vi "CalculateMcsaLowRateFeatures.vi"(5 "Motor Info":T4, 7 "Channel Phasors":T5[](array[typedef]), 8 "error in (no error)":errorcluster, 9 "data flow map in":T10, 10 "waveforms":waveform(sgl)[](array[waveform]), 11 "Channels":T6[](array[typedef])) -> (0 "error out":errorcluster, 2 "Calculation Cache":T1, 3 "Channels":T6[](array[typedef]))   [LabVIEW 2017, in "McsaAnalysisFunctions.lvlib"]
uses:
  <vilib>/addons/InsightCM/Utilities/Analysis/MCSA/McsaAnalysisFunctions.lvlib
  <vilib>/addons/PointValueMap/controls/PointMap.ctl
  <vilib>/addons/InsightCM/Utilities/Analysis/MCSA/controls/McsaChannel.ctl
  <vilib>/addons/InsightCM/Utilities/Analysis/Shared/controls/Feature.ctl
  <vilib>/addons/InsightCM/Utilities/Analysis/Shared/controls/AmplitudeScale.ctl
  <vilib>/addons/InsightCM/MessageBus/Base/controls/KeyValuePair.ctl
  <vilib>/addons/InsightCM/Utilities/Analysis/MCSA/controls/McsaChannelPhasor.ctl
  <vilib>/addons/InsightCM/Utilities/Analysis/MCSA/controls/McsaMotor.ctl
  <vilib>/addons/InsightCM/Utilities/Analysis/MCSA/controls/MotorCalculationCache.ctl
  <vilib>/addons/Electrical Power/Basic/Measurement/subVIs/basic_Power Value.ctl
  <vilib>/addons/InsightCM/Utilities/Analysis/MCSA/controls/TorqueLoadEfficiency.ctl
  <vilib>/addons/InsightCM/Utilities/Analysis/MCSA/controls/PowerSpectrumCalculationCache.ctl
  <vilib>/addons/_NISVFA/_Shared subVIs/Controls/svc_Spectrum Info.ctl
  <vilib>/addons/_NISVFA/_Shared subVIs/Controls/svc_X-Axis Units.ctl
  <vilib>/addons/_NISVFA/_Shared subVIs/Controls/svc_Spectrum Type.ctl
  <vilib>/addons/_NISVFA/_Shared subVIs/Controls/svc_Engineering Units Text Ring.ctl
  <vilib>/addons/_NISVFA/_Shared subVIs/Controls/svc_Weighting Filter Text Ring.ctl
  <vilib>/addons/_NISVFA/_Shared subVIs/Controls/svc_Complimentary Spectrum Units.ctl
  <vilib>/addons/Electrical Power/Basic/NI_EP_Basic.lvlib
  <vilib>/addons/PointValueMap/PointValueMap.lvlib
  <vilib>/addons/InsightCM/Utilities/MCSA/McsaUtilities.lvlib
  <vilib>/addons/InsightCM/Utilities/Analysis/Shared/AnalysisHelper.lvlib
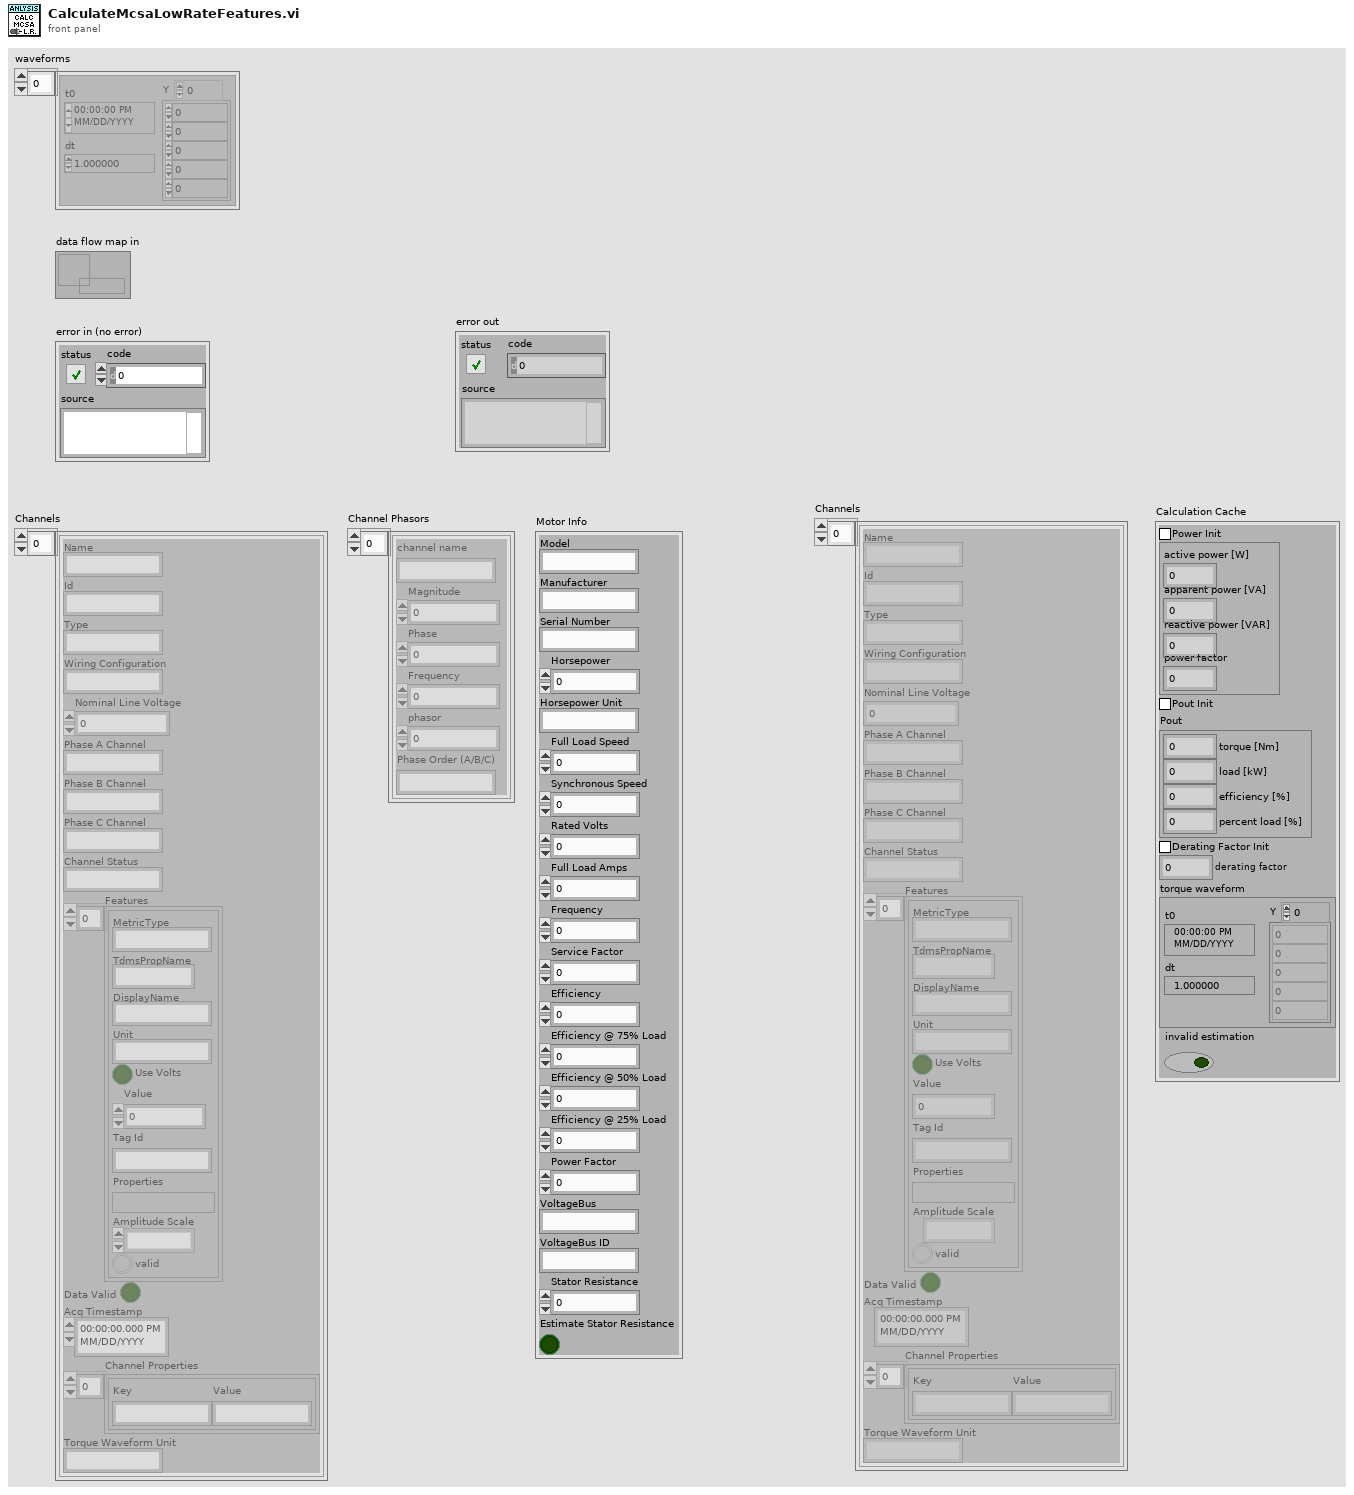
[diagram p1: front panel]
types:
  T1 = typedef "McsaAnalysisFunctions.lvlib/MotorCalculationCache.ctl" = cluster{"Power Init":bool, "power value":T2, "Pout Init":bool, "Pout":T3, "Derating Factor Init":bool, "derating factor":sgl, "torque waveform":waveform(dbl), "invalid estimation":bool}
  T2 = typedef "NI_EP_Basic.lvlib/basic_Power Value.ctl" = cluster{"active power [W]":dbl, "apparent power [VA]":dbl, "reactive power [VAR]":dbl, "power factor":dbl}
  T3 = typedef "McsaAnalysisFunctions.lvlib/TorqueLoadEfficiency.ctl" = cluster{"torque [Nm]":dbl, "load [kW]":dbl, "efficiency [%]":dbl, "percent load [%]":dbl}
  T4 = typedef "McsaAnalysisFunctions.lvlib/McsaMotor.ctl" = cluster{"Model":string, "Manufacturer":string, "Serial Number":string, "Horsepower":dbl, "Horsepower Unit":string, "Full Load Speed":dbl, "Synchronous Speed":dbl, "Rated Volts":dbl, "Full Load Amps":dbl, "Frequency":dbl, "Service Factor":dbl, "Efficiency":dbl, "Efficiency @ 75% Load":dbl, "Efficiency @ 50% Load":dbl, "Efficiency @ 25% Load":dbl, "Power Factor":dbl, "VoltageBus":string, "VoltageBus ID":string, "Stator Resistance":dbl, "Estimate Stator Resistance":bool}
  T5 = typedef "McsaAnalysisFunctions.lvlib/McsaChannelPhasor.ctl" = cluster{"channel name":string, "Magnitude":dbl, "Phase":dbl, "Frequency":dbl, "phasor":cdb, "Phase Order (A/B/C)":string}
  T6 = typedef "McsaAnalysisFunctions.lvlib/McsaChannel.ctl" = cluster{"Name":string, "Id":string, "Type":string, "Wiring Configuration":string, "Nominal Line Voltage":dbl, "Phase A Channel":string, "Phase B Channel":string, "Phase C Channel":string, "Channel Status":string, "Features":T7[], "Data Valid":bool, "Acq Timestamp":timestamp, "Channel Properties":T9[], "Torque Waveform Unit":string}
  T7 = typedef "AnalysisHelper.lvlib/Feature.ctl" = cluster{"MetricType":string, "TdmsPropName":string, "DisplayName":string, "Unit":string, "Use Volts":bool, "Value":dbl, "Tag Id":string, "Properties":variant, "Amplitude Scale":T8, "valid":bool}
  T8 = typedef "AnalysisHelper.lvlib/AmplitudeScale.ctl" = enum16{"rms", "peak", "pk-pk"}
  T9 = typedef "KeyValuePair.ctl" = cluster{"Key":string, "Value":string}
  T10 = typedef "PointValueMap.lvlib/PointMap.ctl" = refnum<data-value>
  T11 = typedef "McsaAnalysisFunctions.lvlib/PowerSpectrumCalculationCache.ctl" = cluster{"Spectrum Init":bool, "Power Spectrum":cluster{"f0":dbl, "df":dbl, "magnitude":dbl[]}, "spectrum info":T12}
  T12 = typedef "svc_Spectrum Info.ctl" = cluster{"channel name":string, "description":string, "x-axis units":T13, "spectral info":cluster{"spectrum type":T14, "linear/dB":enum16{"linear", "dB"}, "window":u16, "window size":i32, "FFT size":i32}, "engineering units":T15, "custom label":string, "dB reference [EU]":dbl, "peak units":enum16{"rms", "peak", "peak-peak"}, "weighting filter":T16, "spectral density?":bool, "unit label":string, "spectrum skewed?":bool, "complimentary spectrum units":T17}
  T13 = typedef "svc_X-Axis Units.ctl" = u16
  T14 = typedef "svc_Spectrum Type.ctl" = enum16{"FFT Spectrum [complex]", "Amplitude [Magnitude]", "Power [Magnitude^2]", "Cross Spectrum [complex]", "Frequency Response [Complex]"}
  T15 = typedef "svc_Engineering Units Text Ring.ctl" = u16
  T16 = typedef "svc_Weighting Filter Text Ring.ctl" = u16
  T17 = typedef "svc_Complimentary Spectrum Units.ctl" = enum16{"none", "radians", "degrees", "cycles", "imaginary"}
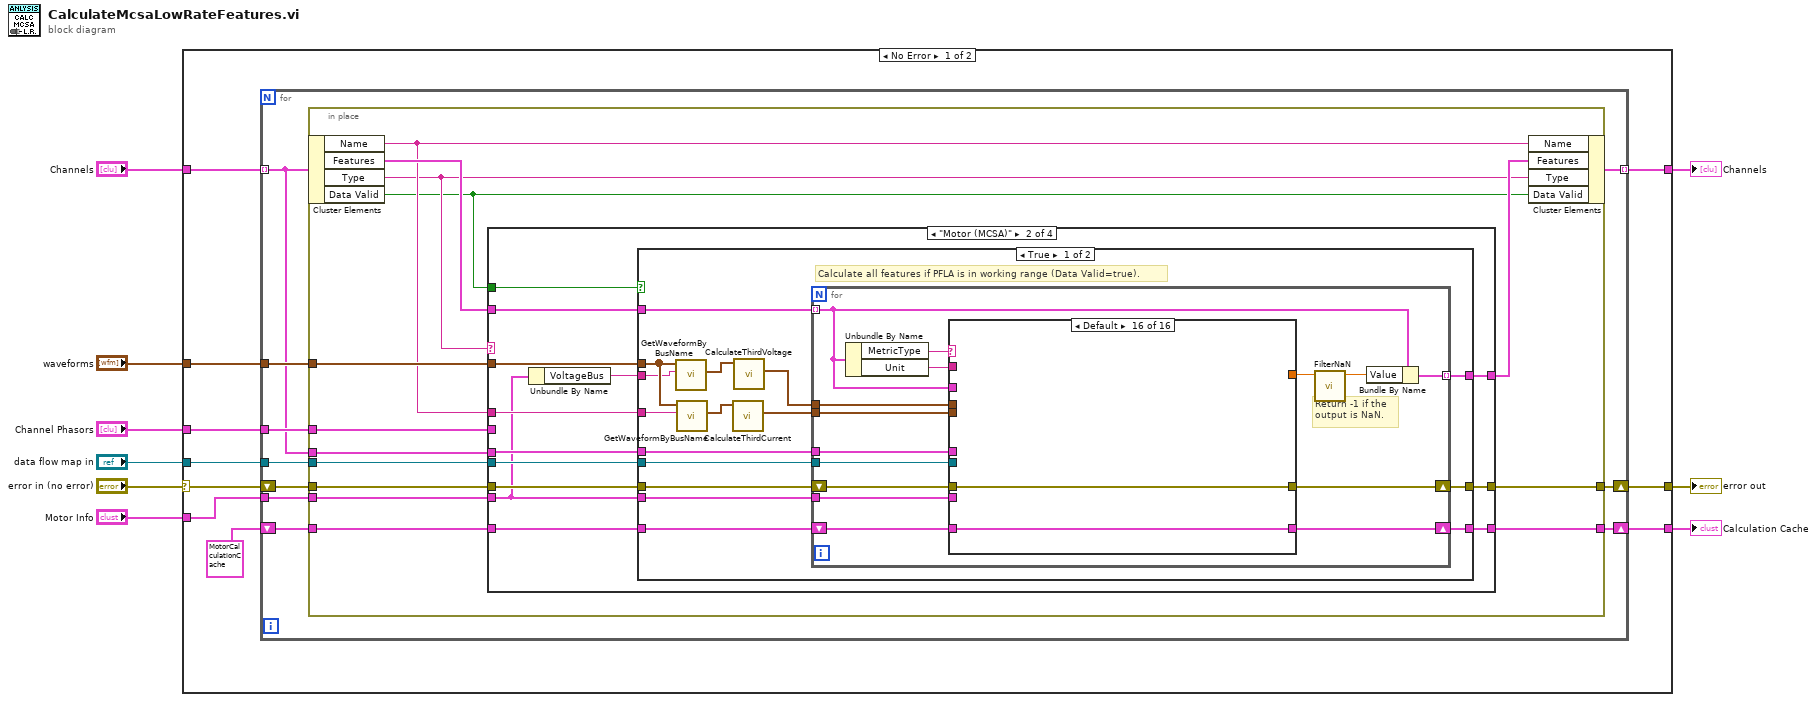
[diagram p0: block diagram]
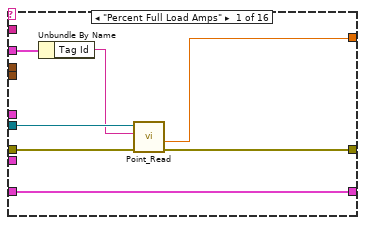
[diagram p3: hidden frame]
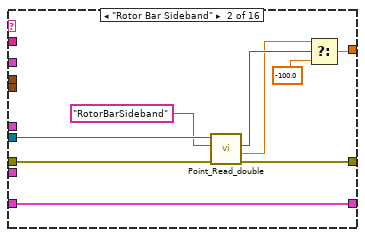
[diagram p4: hidden frame]
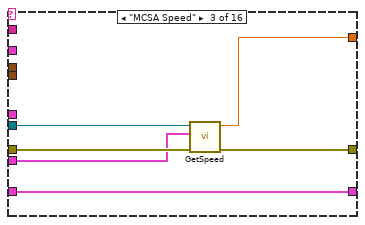
[diagram p5: hidden frame]
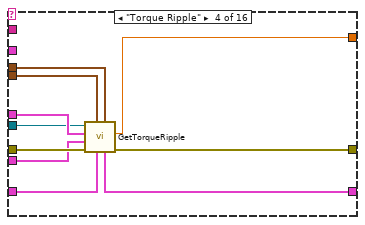
[diagram p6: hidden frame]
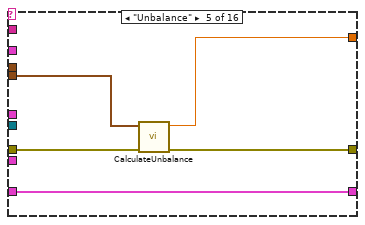
[diagram p7: hidden frame]
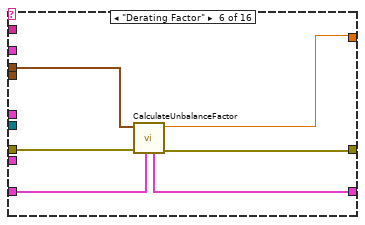
[diagram p8: hidden frame]
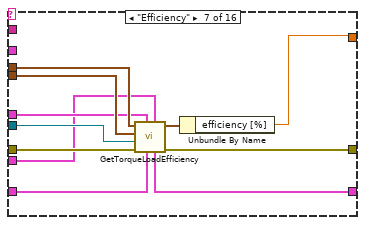
[diagram p9: hidden frame]
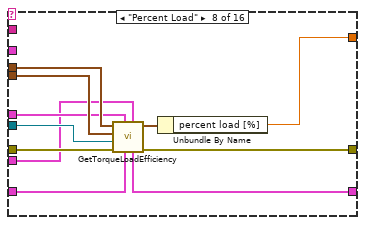
[diagram p10: hidden frame]
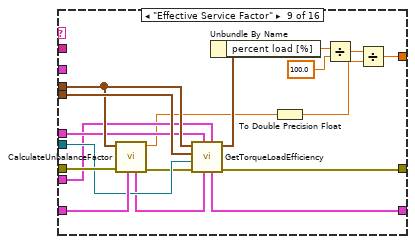
[diagram p11: hidden frame]
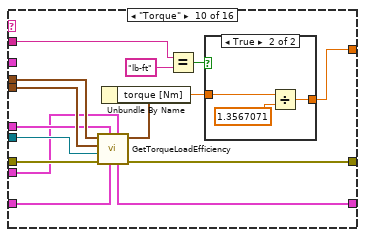
[diagram p12: hidden frame]
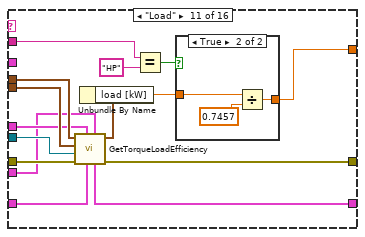
[diagram p14: hidden frame]
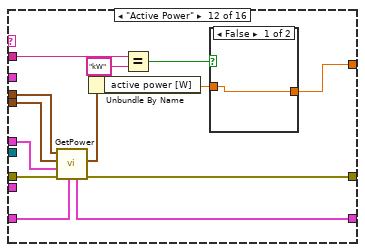
[diagram p16: hidden frame]
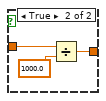
[diagram p17: hidden frame]
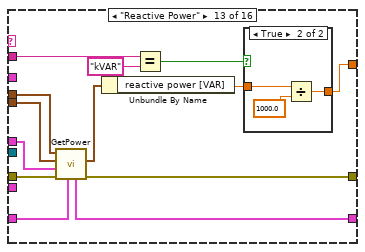
[diagram p18: hidden frame]
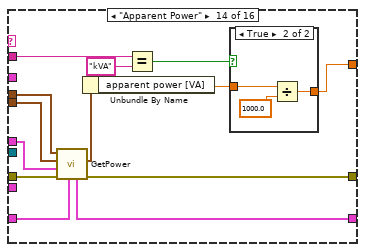
[diagram p20: hidden frame]
diagram:
  n1 = case shown="No Error" "error in (no error)" {
    selector: "error in (no error)" -> [w19 w402]
    tunnel: [w17 w402] -> w9
    tunnel: "waveforms" -> [w18 _]
    tunnel: "data flow map in" -> [w16 _]
    tunnel: "Channels" -> [w15 w401]
    tunnel: [w14 w401] -> w4
    tunnel: "Channel Phasors" -> [w13 _]
    tunnel: "Motor Info" -> [w12 _]
    tunnel: [w11 _] -> w1
    frame No Error {
      n2 = for {
        tunnel: w15 -> [w22] mode=indexing
        tunnel: [w29] -> w14 mode=indexing
        tunnel: w18 -> [w26]
        shift-right: [w27] -> w17
        shift-left: w19 -> [w28]
        tunnel: w16 -> [w25]
        tunnel: w13 -> [w24]
        tunnel: w12 -> [w23]
        shift-right: [w20] -> w11
        shift-left: T1 {"Power Init"=FALSE, "power value"={"active power [W]"=0.0, "apparent power [VA]"=0.0, "reactive power [VAR]"=0.0, "power factor"=0.0}, "Pout Init"=FALSE, "Pout"={"torque [Nm]"=0.0, "load [kW]"=0.0, "efficiency [%]"=0.0, "percent load [%]"=0.0}, "Derating Factor Init"=FALSE, "derating factor"=0.0, "torque waveform"={"t0"=timestamp(0 s since 1904-01-01), "dt"=1.0, "Y"=[]}, "invalid estimation"=FALSE} ("Calculation State in") -> [w21]
        n3 = in-place {
          in-place-border: w28 -> [w40]
          in-place-border: [w43] -> w27
          in-place-border: w26 -> [w39]
          in-place-border: w23 -> [w33]
          in-place-border: w25 -> [w36]
          in-place-border: w24 -> [w35]
          in-place-border: w22 -> [w32]
          in-place-border: w21 -> [w31]
          in-place-border: [w30] -> w20
          n4 = in-place-cluster #1(w22) -> ("Name"=w38:string, "Features"=w42:T7[], "Type"=w37:string, "Data Valid"=w34:bool)
          n5 = case shown="\"Motor (MCSA)\"" w37 {
            tunnel: [w45 w59 w325 w380] -> w41
            tunnel: w40 -> [w46 w53 w324 w373]
            tunnel: w42 -> [w45 w58 w323 w379]
            tunnel: w39 -> [_ w55 w318 w377]
            tunnel: [w46 w57 w322 w378] -> w43
            tunnel: w33 -> [_ w50 w321 _]
            tunnel: w38 -> [_ w56 w315 w376]
            tunnel: w36 -> [_ w54 w320 w374]
            tunnel: w35 -> [_ _ w319 _]
            tunnel: w34 -> [_ w52 _ _]
            tunnel: w32 -> [_ w51 _ _]
            tunnel: w31 -> [w44 w48 w314 w372]
            tunnel: [w44 w47 w314 w372] -> w30
            frame Default {
            }
            frame "Motor (MCSA)" {
              n6 = Unbundle By Name(w50) -> ("VoltageBus"=w49:string)
              n7 = case shown="True" w52 {
                tunnel: [w75 w286] -> w59
                tunnel: w58 -> [w74 w285]
                tunnel: [w73 w284] -> w57
                tunnel: w50 -> [w72 _]
                tunnel: w56 -> [w64 w276]
                tunnel: w55 -> [w69 w281]
                tunnel: w53 -> [w66 w278]
                tunnel: w54 -> [w65 w277]
                tunnel: w51 -> [w63 _]
                tunnel: w49 -> [w62 w275]
                tunnel: w48 -> [w61 w274]
                tunnel: [w60 w274] -> w47
                frame True {
                  # "Calculate all features if PFLA is in working range (Data Valid=true)."
                  n8 = call <vilib>:"GetWaveformByBusName.vi"("Bus Name"=w62, "Acq Waveforms"=w69) -> ("Waveform in ABC Order"=w70:waveform(dbl)[])  [unwired: 7 in, 2 out]
                  n9 = call <vilib>:"GetWaveformByBusName.vi"("Bus Name"=w64, "Acq Waveforms"=w69) -> ("Waveform in ABC Order"=w71:waveform(dbl)[])  [unwired: 7 in, 2 out]
                  n10 = call <vilib>:"CalculateThirdCurrent.vi"("current waveforms in"=w71) -> ("3-phase current waveforms"=w68:waveform(dbl)[])  [unwired: 8 in, 2 out]
                  n11 = call <vilib>:"CalculateThirdVoltage.vi"("voltage waveforms in"=w70) -> ("3-phases voltage waveforms"=w67:waveform(dbl)[])  [unwired: 8 in, 2 out]
                  n12 = for {
                    tunnel: w74 -> [w88] mode=indexing
                    tunnel: [w90] -> w75 mode=indexing
                    tunnel: w72 -> [w89]
                    shift-right: [w78] -> w73
                    shift-left: w66 -> [w80]
                    tunnel: w65 -> [w81]
                    tunnel: w68 -> [w86]
                    shift-right: [w84] -> w60
                    shift-left: w61 -> [w85]
                    tunnel: w67 -> [w83]
                    tunnel: w63 -> [w79]
                    # "Return -1 if the \noutput is NaN."
                    n13 = Unbundle By Name(w88) -> ("MetricType"=w87:string, "Unit"=w82:string)
                    n14 = case shown="Default" w87 {
                      tunnel: [w94 w100 w108 w117 w124 w128 w141 w148 w166 w180 w199 w213 w230 w247 w266 _] -> w77
                      tunnel: w80 -> [w96 w105 w111 w119 w127 w133 w144 w155 w173 w188 w207 w224 w241 w258 w269 w273]
                      tunnel: [w95 w104 w110 w113 w126 w132 w137 w154 w172 w184 w203 w223 w240 w257 w268 w273] -> w78
                      tunnel: w89 -> [_ _ w107 w116 _ _ w135 w146 w164 w178 w197 _ _ _ _ _]
                      tunnel: w88 -> [w93 _ _ _ _ _ _ _ _ _ _ _ _ _ _ _]
                      tunnel: w81 -> [w97 w103 w109 w114 _ _ w138 w153 w167 w187 w206 _ _ _ _ _]
                      tunnel: w86 -> [_ _ _ w121 w125 _ w139 w151 w169 w186 w205 w219 w236 w253 w264 _]
                      tunnel: w85 -> [w91 w106 w112 w120 w123 w131 w143 w150 w171 w183 w202 w222 w239 w256 w271 w272]
                      tunnel: [w91 w106 w112 w118 w123 w130 w142 w149 w170 w182 w201 w221 w238 w255 w270 w272] -> w84
                      tunnel: w83 -> [_ _ _ w122 _ w129 w140 w152 w168 w185 w204 w220 w237 w254 w265 _]
                      tunnel: w82 -> [_ _ _ _ _ _ _ _ _ w181 w200 w215 w232 w249 _ _]
                      tunnel: w79 -> [_ _ _ w115 _ _ w136 w147 w165 w179 w198 w212 w229 w246 w263 _]
                      frame "Percent Full Load Amps" {
                        n15 = Unbundle By Name(w93) -> ("Tag Id"=w92:string)
                        n16 = call-poly <vilib>:"Point_Read.vi"("Error In"=w96, "Tag"=w92, "Map"=w97) -> ("Error Out"=w95:errorcluster, "Value"=w94:dbl)  [unwired: 3 in, 4 out]
                      }
                      frame "Rotor Bar Sideband" {
                        n17 = call <vilib>:"Point_Read_double.vi"("Error In"=w105, "Tag"="RotorBarSideband", "Map"=w103) -> ("Error Out"=w104:errorcluster, "Value"=w101:dbl, "Found?"=w102:bool)  [unwired: 3 in, 3 out]
                        n18 = Select(t=w101, s=w102, f=-100.0) -> (s? t:f=w100:dbl)
                      }
                      frame "MCSA Speed" {
                        n19 = call <vilib>:"GetSpeed.vi"("error in (no error)"=w111, "Motor"=w107, "Map"=w109) -> ("error out"=w110:errorcluster, "Speed [RPM]"=w108:dbl)  [unwired: 7 in]
                      }
                      frame "Torque Ripple" {
                        n20 = call <vilib>:"GetTorqueRipple.vi"("3-phases voltage waveforms"=w122, "Calculation State in"=w120, "3-phase current waveforms"=w121, "error in (no error)"=w119, "Motor info"=w116, "Channel"=w115, "data map"=w114) -> ("error out"=w113:errorcluster, "Torque Ripple (%)"=w117:dbl, "Calculation State out"=w118:T1)  [unwired: 2 out]
                      }
                      frame "Unbalance" {
                        n21 = call <vilib>:"CalculateUnbalance.vi"("error in (no error)"=w127, "3-phase waveforms"=w125) -> ("error out"=w126:errorcluster, "unbalance [%]"=w124:dbl)  [unwired: 8 in]
                      }
                      frame "Derating Factor" {
                        n22 = call <vilib>:"CalculateUnbalanceFactor.vi"("Calculation Cache In"=w131, "error in (no error)"=w133, "voltage waveforms"=w129) -> ("error out"=w132:errorcluster, "derating factor"=w128:sgl, "Calculation Cache Out"=w130:T1)  [unwired: 6 in]
                      }
                      frame "Efficiency" {
                        n23 = call <vilib>:"GetTorqueLoadEfficiency.vi"("Motor Info"=w135, "Calculation State in"=w143, "Channel Config"=w136, "error in (no error)"=w144, "Map"=w138, "current waveform"=w139, "voltage waveform"=w140) -> ("error out"=w137:errorcluster, "Pout"=w134:T3, "Calculation State out"=w142:T1)  [unwired: 2 in]
                        n24 = Unbundle By Name(w134) -> ("efficiency [%]"=w141:dbl)
                      }
                      frame "Percent Load" {
                        n25 = call <vilib>:"GetTorqueLoadEfficiency.vi"("Motor Info"=w146, "Calculation State in"=w150, "Channel Config"=w147, "error in (no error)"=w155, "Map"=w153, "current waveform"=w151, "voltage waveform"=w152) -> ("error out"=w154:errorcluster, "Pout"=w145:T3, "Calculation State out"=w149:T1)  [unwired: 2 in]
                        n26 = Unbundle By Name(w145) -> ("percent load [%]"=w148:dbl)
                      }
                      frame "Effective Service Factor" {
                        n27 = call <vilib>:"CalculateUnbalanceFactor.vi"("Calculation Cache In"=w171, "error in (no error)"=w173, "voltage waveforms"=w168) -> ("error out"=w161:errorcluster, "derating factor"=w162:sgl, "Calculation Cache Out"=w157:T1)  [unwired: 6 in]
                        n28 = call <vilib>:"GetTorqueLoadEfficiency.vi"("Motor Info"=w164, "Calculation State in"=w157, "Channel Config"=w165, "error in (no error)"=w161, "Map"=w167, "current waveform"=w169, "voltage waveform"=w168) -> ("error out"=w172:errorcluster, "Pout"=w163:T3, "Calculation State out"=w170:T1)  [unwired: 2 in]
                        n29 = Unbundle By Name(w163) -> ("percent load [%]"=w160:dbl)
                        n30 = To Double Precision Float(number=w162) -> (double precision float=w156:dbl)
                        n31 = Divide(x=w160, y=100.0) -> (x/y=w159:dbl)
                        n32 = Divide(x=w159, y=w156) -> (x/y=w166:dbl)
                      }
                      frame "Torque" {
                        n33 = call <vilib>:"GetTorqueLoadEfficiency.vi"("Motor Info"=w178, "Calculation State in"=w183, "Channel Config"=w179, "error in (no error)"=w188, "Map"=w187, "current waveform"=w186, "voltage waveform"=w185) -> ("error out"=w184:errorcluster, "Pout"=w174:T3, "Calculation State out"=w182:T1)  [unwired: 2 in]
                        n34 = Unbundle By Name(w174) -> ("torque [Nm]"=w177:dbl)
                        n35 = Equal?(x=w181, y="lb-ft") -> (x = y?=w175:bool)
                        n36 = case shown="True" w175 {
                          tunnel: w177 -> [w189 w190]
                          tunnel: [w189 w192] -> w180
                          frame False {
                          }
                          frame True {
                            n37 = Divide(x=w190, y=1.3567071) -> (x/y=w192:dbl)
                          }
                        }
                      }
                      frame "Load" {
                        n38 = call <vilib>:"GetTorqueLoadEfficiency.vi"("Motor Info"=w197, "Calculation State in"=w202, "Channel Config"=w198, "error in (no error)"=w207, "Map"=w206, "current waveform"=w205, "voltage waveform"=w204) -> ("error out"=w203:errorcluster, "Pout"=w193:T3, "Calculation State out"=w201:T1)  [unwired: 2 in]
                        n39 = Unbundle By Name(w193) -> ("load [kW]"=w196:dbl)
                        n40 = Equal?(x=w200, y="HP") -> (x = y?=w194:bool)
                        n41 = case shown="True" w194 {
                          tunnel: w196 -> [w208 w209]
                          tunnel: [w208 w211] -> w199
                          frame False {
                          }
                          frame True {
                            n42 = Divide(x=w209, y=0.7457) -> (x/y=w211:dbl)
                          }
                        }
                      }
                      frame "Active Power" {
                        n43 = call <vilib>:"GetPower.vi"("Calculation State in"=w222, "error in (no error)"=w224, "Channel"=w212, "3-phase current waveform"=w219, "3-phase voltage waveform"=w220) -> ("error out"=w223:errorcluster, "power value"=w214:T2, "Calculation State out"=w221:T1)  [unwired: 4 in]
                        n44 = Unbundle By Name(w214) -> ("active power [W]"=w218:dbl)
                        n45 = Equal?(x=w215, y="kW") -> (x = y?=w217:bool)
                        n46 = case shown="False" w217 {
                          tunnel: w218 -> [w225 w228]
                          tunnel: [w225 w227] -> w213
                          frame False {
                          }
                          frame True {
                            n47 = Divide(x=w228, y=1000.0) -> (x/y=w227:dbl)
                          }
                        }
                      }
                      frame "Reactive Power" {
                        n48 = call <vilib>:"GetPower.vi"("Calculation State in"=w239, "error in (no error)"=w241, "Channel"=w229, "3-phase current waveform"=w236, "3-phase voltage waveform"=w237) -> ("error out"=w240:errorcluster, "power value"=w231:T2, "Calculation State out"=w238:T1)  [unwired: 4 in]
                        n49 = Unbundle By Name(w231) -> ("reactive power [VAR]"=w235:dbl)
                        n50 = Equal?(x=w232, y="kVAR") -> (x = y?=w234:bool)
                        n51 = case shown="True" w234 {
                          tunnel: w235 -> [w242 w245]
                          tunnel: [w242 w244] -> w230
                          frame False {
                          }
                          frame True {
                            n52 = Divide(x=w245, y=1000.0) -> (x/y=w244:dbl)
                          }
                        }
                      }
                      frame "Apparent Power" {
                        n53 = call <vilib>:"GetPower.vi"("Calculation State in"=w256, "error in (no error)"=w258, "Channel"=w246, "3-phase current waveform"=w253, "3-phase voltage waveform"=w254) -> ("error out"=w257:errorcluster, "power value"=w248:T2, "Calculation State out"=w255:T1)  [unwired: 4 in]
                        n54 = Unbundle By Name(w248) -> ("apparent power [VA]"=w252:dbl)
                        n55 = Equal?(x=w249, y="kVA") -> (x = y?=w251:bool)
                        n56 = case shown="True" w251 {
                          tunnel: w252 -> [w259 w262]
                          tunnel: [w259 w261] -> w247
                          frame False {
                          }
                          frame True {
                            n57 = Divide(x=w262, y=1000.0) -> (x/y=w261:dbl)
                          }
                        }
                      }
                      frame "Power Factor" {
                        n58 = call <vilib>:"GetPower.vi"("Calculation State in"=w271, "error in (no error)"=w269, "Channel"=w263, "3-phase current waveform"=w264, "3-phase voltage waveform"=w265) -> ("error out"=w268:errorcluster, "power value"=w267:T2, "Calculation State out"=w270:T1)  [unwired: 4 in]
                        n59 = Unbundle By Name(w267) -> ("power factor"=w266:dbl)
                      }
                      frame Default {
                      }
                    }
                    n60 = call <vilib>:"FilterNaN.vi"("input value"=w77) -> ("filtered value"=w76:dbl)  [unwired: 10 in]
                    n61 = Bundle By Name(cluster=w88, "Value"=w76) -> (w90:T7)
                  }
                }
                frame False {
                  n62 = call <vilib>:"GetWaveformByBusName.vi"("Bus Name"=w275, "Acq Waveforms"=w281) -> ("Waveform in ABC Order"=w282:waveform(dbl)[])  [unwired: 7 in, 2 out]
                  n63 = call <vilib>:"GetWaveformByBusName.vi"("Bus Name"=w276, "Acq Waveforms"=w281) -> ("Waveform in ABC Order"=w283:waveform(dbl)[])  [unwired: 7 in, 2 out]
                  n64 = call <vilib>:"CalculateThirdCurrent.vi"("current waveforms in"=w283) -> ("3-phase current waveforms"=w280:waveform(dbl)[])  [unwired: 8 in, 2 out]
                  n65 = call <vilib>:"CalculateThirdVoltage.vi"("voltage waveforms in"=w282) -> ("3-phases voltage waveforms"=w279:waveform(dbl)[])  [unwired: 8 in, 2 out]
                  n66 = for {
                    tunnel: w285 -> [w292] mode=indexing
                    tunnel: [w295] -> w286 mode=indexing
                    shift-right: [w294] -> w284
                    shift-left: w278 -> [w288]
                    tunnel: w280 -> [w290]
                    tunnel: w279 -> [w289]
                    tunnel: w277 -> [w287]
                    n67 = Unbundle By Name(w292) -> ("MetricType"=w291:string)
                    n68 = case shown="\"Percent Full Load Amps\"" w291 {
                      tunnel: [w298 w305 w308 0.0 ("power factor")] -> w293
                      tunnel: w288 -> [w300 w302 w311 w313]
                      tunnel: [w299 w306 w310 w313] -> w294
                      tunnel: w292 -> [w297 _ _ _]
                      tunnel: w287 -> [w301 w303 w309 _]
                      tunnel: w290 -> [_ _ _ _]
                      tunnel: w289 -> [_ _ _ _]
                      frame "Percent Full Load Amps" {
                        # "Only update PFLA if out of range."
                        n69 = Unbundle By Name(w297) -> ("Tag Id"=w296:string)
                        n70 = call-poly <vilib>:"Point_Read.vi"("Error In"=w300, "Tag"=w296, "Map"=w301) -> ("Error Out"=w299:errorcluster, "Value"=w298:dbl)  [unwired: 3 in, 4 out]
                      }
                      frame "MCSA Speed" {
                        w305 = 0.0 ("power factor")
                        # "Set the default value if PFLA is out of range."
                        n71 = call <vilib>:"Point_Write_double.vi"("Error In"=w302, "Value"=w305, "Tag"="Speed", "Map"=w303) -> ("Error Out"=w306:errorcluster)  [unwired: 6 in, 1 out]
                      }
                      frame "Rotor Bar Sideband" {
                        w308 = -100.0 ("power factor")
                        # "Set the default value if PFLA is out of range."
                        n72 = call <vilib>:"Point_Write_double.vi"("Error In"=w311, "Value"=w308, "Tag"="RotorBarSideband", "Map"=w309) -> ("Error Out"=w310:errorcluster)  [unwired: 6 in, 1 out]
                      }
                      frame Default {
                      }
                    }
                    n73 = Bundle By Name(cluster=w292, "Value"=w293) -> (w295:T7)
                  }
                }
              }
            }
            frame "NI 9239 MCSA", "NI 9242 MCSA" {
              n74 = call <vilib>:"GetWaveformByName.vi"("Channel Name"=w315, "Acq Waveforms"=w318) -> ("Waveform"=w317:waveform(sgl))  [unwired: 6 in, 3 out]
              n75 = for {
                tunnel: w323 -> [w332] mode=indexing
                tunnel: [w338] -> w325 mode=indexing
                tunnel: w317 -> [w334]
                tunnel: w321 -> [w333]
                shift-right: [w336] -> w322
                shift-left: w324 -> [w337]
                tunnel: w315 -> [w330]
                tunnel: w320 -> [w329]
                tunnel: w319 -> [w328]
                shift-right: [w327] -> _
                shift-left: T11 {"Spectrum Init"=FALSE, "Power Spectrum"={"f0"=0.0, "df"=0.0, "magnitude"=[]}, "spectrum info"={"channel name"="", "description"="", "x-axis units"=0, "spectral info"={"spectrum type"=enum."Power [Magnitude^2]", "linear/dB"=enum."linear", "window"=0, "window size"=0, "FFT size"=0}, "engineering units"=0, "custom label"="", "dB reference [EU]"=0.0, "peak units"=enum."rms", "weighting filter"=0, "spectral density?"=FALSE, "unit label"="", "spectrum skewed?"=FALSE, "complimentary spectrum units"=enum."none"}} ("Calculation State out") -> [w326]
                n76 = Unbundle By Name(w332) -> ("MetricType"=w331:string)
                n77 = case shown="\"MCSA RMS\"" w331 {
                  tunnel: [w340 w347 w354 w365 _] -> w335
                  tunnel: w337 -> [w345 w352 w358 w369 w371]
                  tunnel: [w344 w351 w357 w368 w371] -> w336
                  tunnel: w334 -> [_ _ _ w367 _]
                  tunnel: w333 -> [_ _ _ w360 _]
                  tunnel: w332 -> [_ _ w355 w366 _]
                  tunnel: w330 -> [w342 w349 _ _ _]
                  tunnel: w329 -> [_ _ w356 w364 _]
                  tunnel: w328 -> [w343 w350 _ _ _]
                  tunnel: [w339 w346 w353 w362 w370] -> w327
                  tunnel: w326 -> [w339 w346 w353 w361 w370]
                  frame "Phasor: Magnitude" {
                    n78 = call <vilib>:"GetPhasorByChannelName.vi"("error in (no error)"=w345, "Channel Name"=w342, "Channels Phasor"=w343) -> ("error out"=w344:errorcluster, "Channel Phasor"=w341:T5)  [unwired: 6 in, 1 out]
                    n79 = Unbundle By Name(w341) -> ("Magnitude"=w340:dbl)
                  }
                  frame "Phasor: Phase" {
                    n80 = call <vilib>:"GetPhasorByChannelName.vi"("error in (no error)"=w352, "Channel Name"=w349, "Channels Phasor"=w350) -> ("error out"=w351:errorcluster, "Channel Phasor"=w348:T5)  [unwired: 6 in, 1 out]
                    n81 = Unbundle By Name(w348) -> ("Phase"=w347:dbl)
                  }
                  frame "MCSA RMS" {
                    n82 = Unbundle By Name(w355) -> ("Tag Id"=w359:string)
                    n83 = call-poly <vilib>:"Point_Read.vi"("Error In"=w358, "Tag"=w359, "Map"=w356) -> ("Error Out"=w357:errorcluster, "Value"=w354:dbl)  [unwired: 3 in, 4 out]
                  }
                  frame "Spectral Band", "Spectral Band: Orders", "Spectral Band: Phase" {
                    n84 = call <vilib>:"GetSpeed.vi"("Motor"=w360, "Map"=w364) -> ("Speed [RPM]"=w363:dbl)  [unwired: 8 in, 1 out]
                    n85 = call <vilib>:"CalculateBand.vi"("Waveform"=w367, "Feature"=w366, "Speed [RPM]"=w363, "error in (no error)"=w369, "Calculation State in"=w361) -> ("Band Value"=w365:sgl, "Calculation State out"=w362:T11, "error out"=w368:errorcluster)  [unwired: 8 in]
                  }
                  frame Default {
                  }
                }
                n86 = Bundle By Name(cluster=w332, "Value"=w335) -> (w338:T7)
              }
            }
            frame "Voltage Bus" {
              n87 = call <vilib>:"GetWaveformByBusName.vi"("Bus Name"=w376, "Acq Waveforms"=w377) -> ("Waveform in ABC Order"=w375:waveform(dbl)[])  [unwired: 7 in, 2 out]
              n88 = for {
                tunnel: w379 -> [w383] mode=indexing
                tunnel: [w388] -> w380 mode=indexing
                tunnel: w375 -> [w384]
                shift-right: [w386] -> w378
                shift-left: w373 -> [w387]
                tunnel: w374 -> [w381]
                n89 = Unbundle By Name(w383) -> ("MetricType"=w382:string)
                n90 = case shown="Default" w382 {
                  tunnel: [w389 w395 _] -> w385
                  tunnel: w387 -> [w392 w397 w400]
                  tunnel: [w393 w396 w400] -> w386
                  tunnel: w384 -> [w391 w394 _]
                  tunnel: w383 -> [_ _ _]
                  tunnel: w381 -> [w390 _ _]
                  frame "Line Frequency" {
                    n91 = call <vilib>:"GetFreq.vi"("error in (no error)"=w392, "Map"=w390, "waveforms"=w391) -> ("error out"=w393:errorcluster, "frequency"=w389:dbl)  [unwired: 7 in]
                  }
                  frame "Unbalance" {
                    n92 = call <vilib>:"CalculateThirdVoltage.vi"("error out"=w397, "voltage waveforms in"=w394) -> ("error out"=w399:errorcluster, "3-phases voltage waveforms"=w398:waveform(dbl)[])  [unwired: 7 in, 1 out]
                    n93 = call <vilib>:"CalculateUnbalance.vi"("error in (no error)"=w399, "3-phase waveforms"=w398) -> ("error out"=w396:errorcluster, "unbalance [%]"=w395:dbl)  [unwired: 8 in]
                  }
                  frame Default {
                  }
                }
                n94 = Bundle By Name(cluster=w383, "Value"=w385) -> (w388:T7)
              }
            }
          }
          n95 = in-place-cluster #1("Name"=w38, "Features"=w41, "Type"=w37, "Data Valid"=w34) -> (w29:T6)
        }
      }
    }
    frame Error {
    }
  }
  "error out" <- w9
  "Channels" <- w4
  "Calculation Cache" <- w1
